vi "Terminal-ModbusEthernet-WriteCoil.vi"(5 "write operation timeout (ms)":i32=5000 caption="写操作超时（毫秒）", 7 "read operation timeout (ms)":i32=5000 caption="读操作超时（毫秒）", 8 "error in":errorcluster, 9 "coil value":bool caption="线圈值", 10 "address":u16 caption="地址", 11 "unit ID":u8 caption="单元ID") -> (0 "error out":errorcluster)   [LabVIEW 2014]
uses:
  <vilib>/Modbus/subvis/Modbus API/Modbus API.lvclass/Modbus API.ctl
  <vilib>/Modbus/subvis/Transmission Data Unit (ADU)/Transmission Data Unit/Transmission Data Unit.lvclass/Transmission Data Unit.ctl
  <vilib>/Modbus/master/Data Access/Unit ID/Set Unit ID Property.vi
  <vilib>/Modbus/subvis/Transmission Data Unit (ADU)/Transmission Data Unit/Data Access/Unit ID/Write Unit ID.vi
  <vilib>/Modbus/subvis/Modbus API/Read Transmission Data Unit.vi
  <vilib>/Modbus/subvis/Modbus API/Write Transmission Data Unit.vi
  Configuration-Global.vi
  <vilib>/Modbus/master/Create Master Instance (TCP).vi
  <vilib>/Modbus/subvis/Transmission Data Unit (ADU)/Transmission Data Unit/Transmission Data Unit.lvclass
  <vilib>/Modbus/master/Modbus Master.lvclass
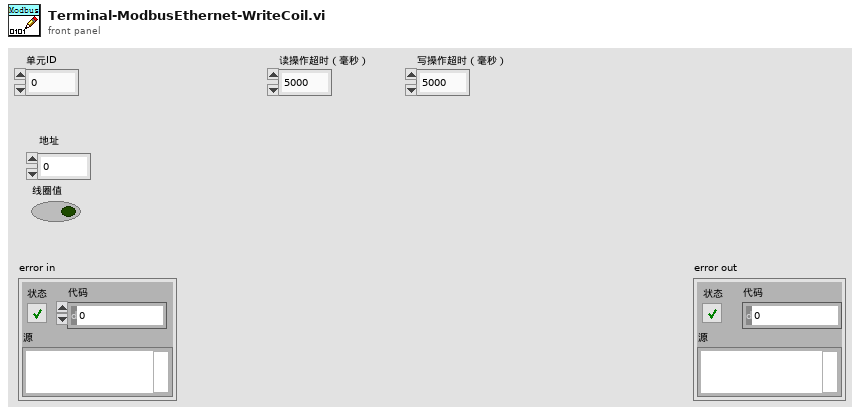
[diagram p1: front panel]
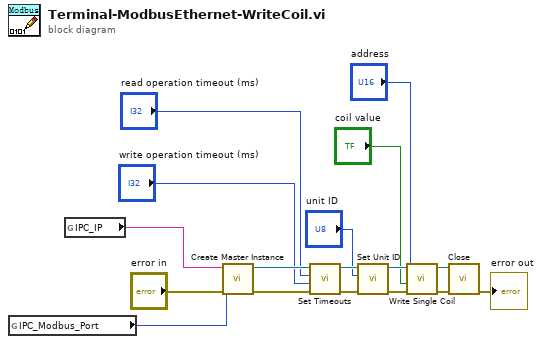
[diagram p0: block diagram]
diagram:
  n1 = global read "Configuration-Global.vi" "IPC_Modbus_Port"() -> (w4:i32)
  n2 = global read "Configuration-Global.vi" "IPC_IP"() -> (w3:string)
  n3 = call-poly <vilib>:"Create Master Instance.vi"("error in (no error)"="error in", "port (502)"=w4, "address"=w3) -> ("error out"=w15:errorcluster, "TCP master instance"=w14:refnum<class "Modbus Master.lvclass">)  [unwired: 7 in]
  n4 = call <vilib>:"Set Timeouts.vi"("error in (no error)"=w15, "write operation timeout (ms)"="write operation timeout (ms)", "read operation timeout (ms)"="read operation timeout (ms)", "Modbus master in"=w14) -> ("error out"=w6:errorcluster, "Modbus master out"=w16:refnum<class "Modbus Master.lvclass">)  [unwired: 6 in]
  n5 = call <vilib>:"Set Unit ID.vi"("error in (no error)"=w6, "unit ID"="unit ID", "Modbus master in"=w16) -> ("error out"=w8:errorcluster, "Modbus master out"=w7:refnum<class "Modbus Master.lvclass">)  [unwired: 7 in]
  n6 = call-dynamic "Write Single Coil.vi"("error in (no error)"=w8, "coil value"="coil value", "address"="address", "Modbus master in"=w7) -> ("error out"=w10:errorcluster, "Modbus master out"=w11:refnum<class "Modbus Master.lvclass">)  [unwired: 6 in]
  n7 = call-dynamic "Close.vi"("error in (no error)"=w10, "Modbus master in"=w11) -> ("error out"=→"error out":errorcluster)  [unwired: 9 in]
